vi "Point&Path@Pallet1D__Parameter.vi"(1 "ParamterIn":string) -> (0 "ParamterOut":string)   [LabVIEW 2020]
panel:
  in  "Number":string(combo)
  in  "PointName":string(combo)
  in  "Confirm":bool
  # "Point&Path@Pallet1D $Point,$Number\n$Point[0]=Start\n$Point[1]=End"
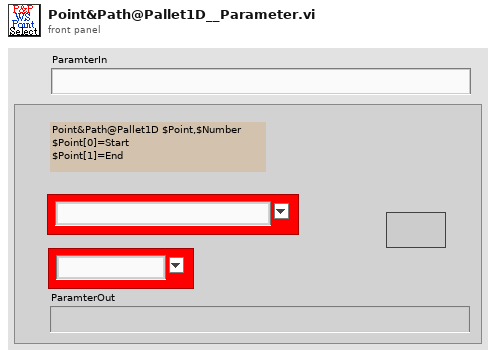
[diagram p1: front panel]
types:
  T1 = enum16{"Get", "UpdatePointS", "Init", "UpdateIndex", "GetCurrent&Index+1", "GetWithIndex", "ChkLast", "GetCurrent"}
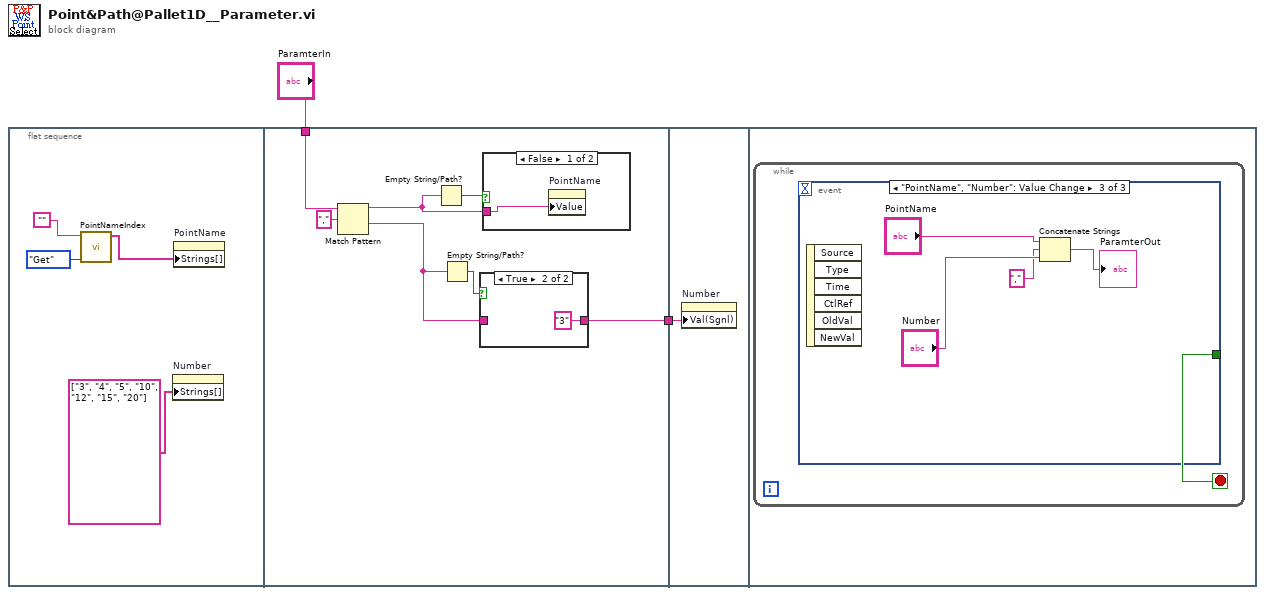
[diagram p0: block diagram]
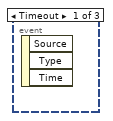
[diagram p4: hidden frame]
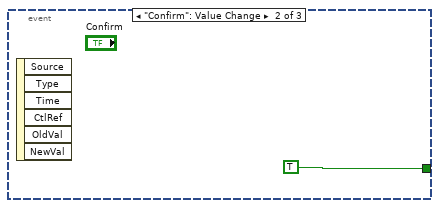
[diagram p5: hidden frame]
diagram:
  n1 = flat-sequence {
    tunnel: "ParamterIn" -> [w10]
    tunnel: [w11] -> w1
    tunnel: w1 -> [w17]
    frame #0 {
      n2 = call "PointNameIndex.vi"("OP"=T1."Get", "PointName"="") -> ("PointNameList"=w4:string[])  [unwired: 4 in, 5 out]
      n3 = property on="Number" class="CmbBox"("Strings[]"=string[] ["3", "4", "5", "10", "12", "15", "20"] ("Strings []")) -> ()  [unwired: 2 in, 2 out]
      n4 = property on="PointName" class="CmbBox"("Strings[]"=w4) -> ()  [unwired: 2 in, 2 out]
    }
    frame #1 {
      n5 = Match Pattern(string=w10, regular expression="," ("search string")) -> (before substring=w7:string, after substring=w8:string)  [unwired: 1 in, 2 out]
      n6 = Empty String/Path?(string/path=w7) -> (empty?=w13:bool)
      n7 = Empty String/Path?(string/path=w8) -> (empty?=w12:bool)
      n8 = case shown="True" w12 {
        tunnel: [w14 "3" ("ParamterIn")] -> w11
        tunnel: w8 -> [w14 _]
        frame False {
        }
        frame True {
        }
      }
      n9 = case shown="False" w13 {
        tunnel: w7 -> [w16 _]
        frame False {
          n10 = property on="PointName" class="CmbBox"("Value"=w16) -> ()  [unwired: 2 in, 2 out]
        }
        frame True {
        }
      }
    }
    frame #2 {
      n11 = property on="Number" class="CmbBox"("Val(Sgnl)"=w17) -> ()  [unwired: 2 in, 2 out]
    }
    frame #3 {
      n12 = while {
        stop <- w18 stop-if-true
        n13 = event shown="[2] \"PointName\", \"Number\": Value Change" {
          selector: _ -> [_ _ _]
          dyn-events: _ -> [_ _ _]
          timeout: _ -> [_ _ _]
          tunnel: [_ TRUE _] -> w18
          event Timeout {
            n14 = event-data() -> ()  [unwired: 1 in, 3 out]
          }
          event "Confirm": Value Change {
            n15 = event-data() -> ()  [unwired: 1 in, 6 out]
          }
          event "PointName", "Number": Value Change {
            n16 = event-data() -> ()  [unwired: 1 in, 6 out]
            n17 = Concatenate Strings("PointName", ",", "Number") -> (→"ParamterOut":string)
          }
        }
      }
    }
  }
